vi "GermanInfo_Select_actual_values.vi"(11 "CSMinfo in":T1={"Общие сведения"={"Регистрационный номер заказа"="", "Идентификация (шифр) образца"="", "IMEI образца"="", "НД, устанавливающий требования"="", "Методы испытаний (измерений)"="", "Дата начала испытаний"="", "Дата завершения испытаний"=""}, "Климатические условия внешней среды"={"Температура окружающего воздуха"="", "Относительная влажность воздуха"="", "Атмосферное давление"=""}, "Окно с настройками"={"Режим звонка связь"=0, "Напряжение источника"=0, "Условия окружающей среды"=0, "Номер образца"=0, "Источник питания"=0, "Номер испытания"=0, "Режим звонка тональный модем"=0, "Количество итераций TM"=100.0, "Аутентификация"=0, "Колличество повторов измерений"=1.0, "Сим карта"=0, "VISA adress of CMW500"="", "Input attenuation"=1.0, "Output attenuation"=1.0, "Call Release Type"=0, "GSM Band"=0, "BCCH Channel Number"=0.0, "TCH Channel Number"=0.0, "Codec"=0, "AWGN"=0, "snrRatioInDb"=0.0, "GSM Fading"=0, "UL C/I ratio"=0, "Use a custom network ID"=FALSE, "MCC (Mobile Country Code)"=0.0, "MNC (Mobile Network Code)"=0.0, "NCC (Network Color Code)"=0.0, "MNC digit count"=0, "BCC (Base station Color Code)"=0.0, "LAC (Location Area Code)"=0.0, "RAC (Routing Area Code)"=0.0, "Cell Identity"=0.0, "Override UE ID"=FALSE, "MCC (UE Mobile Country Code)"=0.0, "MNC (UE Mobile Network Code)"=0.0, "MSIN (Mobile Subscription ID)"=0.0, "InputScaleFactor"=0, "OutputScaleFactor"=0, "Post MSD wave file playback 3GPP  26.269 \nEU_DTMF_tones"=FALSE, "Scenario"=0, "AlAckBehavior"=0, "PSAP listens for PUSH"=FALSE, "BCCH Channel Power"=0.0, "TCH Channel Power"=0.0, "Setting Path"=path "", "Алгоритм дозвона"=0}} {"Окно с настройками"."Алгоритм дозвона" items=["Standart", "Recall"]; "Окно с настройками"."AlAckBehavior" items=["POSITIVE", "CLEAR_DOWN", "LOOP_BACK_MSD_PART"]; "Окно с настройками"."Scenario" items=["NORMAL", "NORMAL_IMMEDIATE_START", "TIMEOUT_T3", "ALLRV_REQ", "SUPPRESS_MSD", "SUPPRESS_ALACK", "SUPPRESS_SEND_MSD"]; "Окно с настройками"."OutputScaleFactor" items=["ONE", "QUARTER", "HALF", "TWO", "FOUR"]; "Окно с настройками"."InputScaleFactor" items=["ONE", "QUARTER", "HALF", "TWO", "FOUR"]; "Окно с настройками"."MNC digit count" items=["TWO", "THREE"]; "Окно с настройками"."UL C/I ratio" items=["Ci1Db", "Ci4Db", "Ci7Db", "Ci10Db", "Ci13Db", "Ci16Db"]; "Окно с настройками"."GSM Fading" items=["GsmFadingOff", "GsmEtsiTs103412DlFading", "GsmEtsiTs103412UlFading", "GsmEtsiTs103412DlUlFading"]; "Окно с настройками"."AWGN" items=["Off", "50MhzAwgn"]; "Окно с настройками"."Codec" items=["FRV2", "AMRH_GMSK_7K95", "AMRH_GMSK_7K40", "AMRH_GMSK_6K70", "AMRH_GMSK_5K90", "AMRH_GMSK_5K15", "AMRH_GMSK_4K75", "AMRF_GMSK_12K20", "AMRF_GMSK_10K20", "AMRF_GMSK_7K95", "AMRF_GMSK_7K40 ", "AMRF_GMSK_6K70", "AMRF_GMSK_5K90", "AMRF_GMSK_5K15", "AMRF_GMSK_4K75", "FRV1", "HRV1", "WAMR_GMSK_6K60", "WAMR_GMSK_8K85", "WAMR_GMSK_12K65"]; "Окно с настройками"."GSM Band" items=["GSM450", "GSM850", "GSM900", "GSM1800", "GSM1900"]; "Окно с настройками"."Call Release Type" items=["NormalRelease", "CallInterruption"]; "Окно с настройками"."Сим карта" items=["SIM", "eSIM"]; "Окно с настройками"."Колличество повторов измерений" min=1.0 max=100.0 format="%#_3g"; "Окно с настройками"."Аутентификация" items=["On", "Off"]; "Окно с настройками"."Режим звонка тональный модем" items=["Автоматически (AT) GEMALTO", "Автоматически (AT) SIMCOM", "Автоматически (AT) SIMCOM SIM7600E-H", "Автоматически (AT) TELIT", "Автоматически (AT) PROGRESS", "Автоматически (AT) PROGRESS GREEN", "Автоматически (AT) PROGRESS BLUE", "Автоматически (реле)", "Вручную"]; "Окно с настройками"."Номер испытания" items=["1", "2", "3"]; "Окно с настройками"."Источник питания" items=["Не используется", "IT6332A"]; "Окно с настройками"."Номер образца" items=["1", "2", "3"]; "Окно с настройками"."Условия окружающей среды" items=["UnormTnorm", "UminTmin", "UmaxTmin", "UminTmax", "UmaxTmax", "TypeA", "TypeB"]; "Окно с настройками"."Напряжение источника" items=["12", "24"]; "Окно с настройками"."Режим звонка связь" items=["Автоматически (AT) GEMALTO", "Автоматически (AT) SIMCOM", "Автоматически (AT) SIMCOM SIM7600E-H", "Автоматически (AT) TELIT", "Автоматически (AT) PROGRESS", "Автоматически (AT) PROGRESS GREEN", "Автоматически (AT) PROGRESS BLUE", "Автоматически (реле)", "Вручную"]}) -> (0 "Условия окружающей среды":u16, 1 "Напряжение источника":u16, 2 "Образец":u16, 3 "Режим звонка":u16)   [LabVIEW 2018]
uses:
  CSM MOSCOW/CSMinfo/data/CSMinfo.ctl
panel:
  # "1. Общие настройки"
  # "Настройки модема по умолчанию"
  # "CMW500"
  # "PSAP"
  # "8.6.6"
  # "8.6.7"
  # "GSM"
  # "2. Настройки связи"
  # "8.6.8 (Use parameter NORMAL_IMMEDIATE_START)"
  # "8.6.9 (Use parameter LOOP_BACK_MSD_PART)"
  # "8.6.6"
  # "3. Настройки тонального модема"
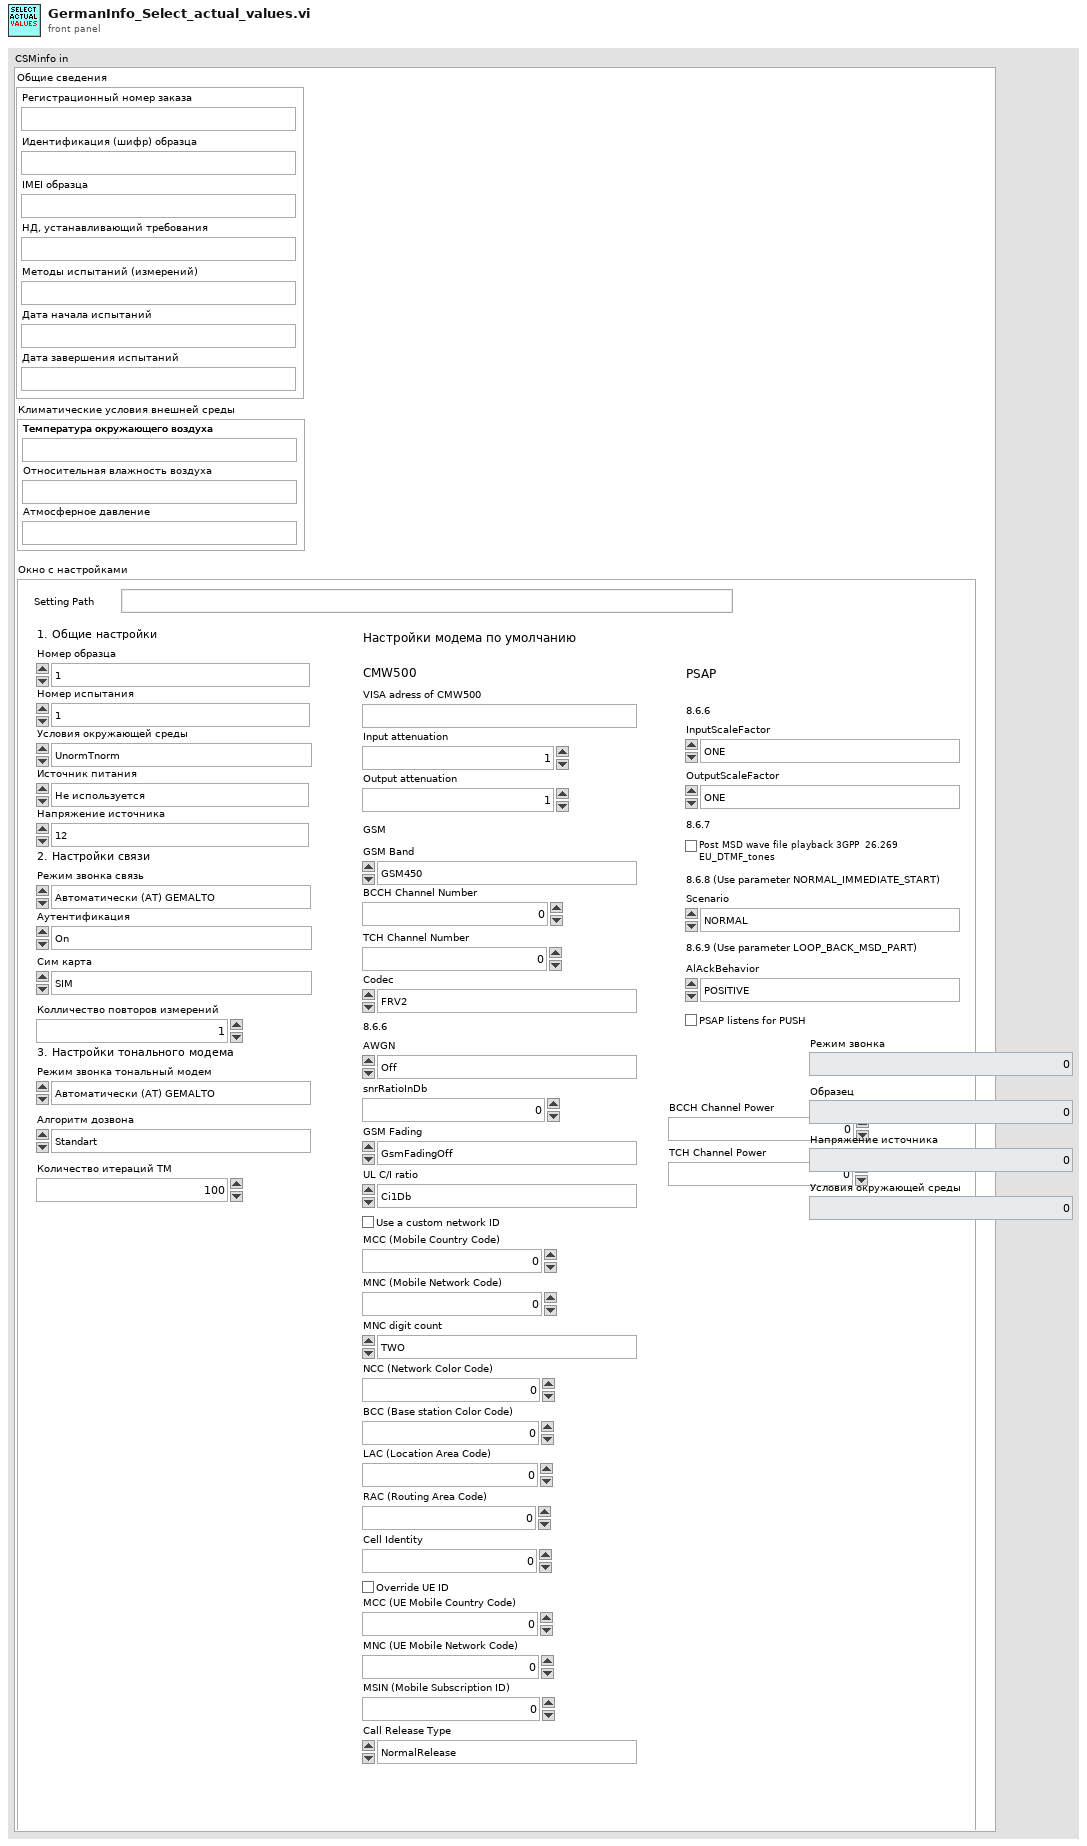
[diagram p1: front panel]
types:
  T1 = typedef "CSMinfo.ctl" = cluster{"Общие сведения":cluster{"Регистрационный номер заказа":string, "Идентификация (шифр) образца":string, "IMEI образца":string, "НД, устанавливающий требования":string, "Методы испытаний (измерений)":string, "Дата начала испытаний":string, "Дата завершения испытаний":string}, "Климатические условия внешней среды":cluster{"Температура окружающего воздуха":string, "Относительная влажность воздуха":string, "Атмосферное давление":string}, "Окно с настройками":cluster{"Режим звонка связь":u16, "Напряжение источника":u16, "Условия окружающей среды":u16, "Номер образца":u16, "Источник питания":u16, "Номер испытания":u16, "Режим звонка тональный модем":u16, "Количество итераций TM":dbl, "Аутентификация":u16, "Колличество повторов измерений":dbl, "Сим карта":u16, "VISA adress of CMW500":string, "Input attenuation":dbl, "Output attenuation":dbl, "Call Release Type":u16, "GSM Band":u16, "BCCH Channel Number":dbl, "TCH Channel Number":dbl, "Codec":u16, "AWGN":u16, "snrRatioInDb":dbl, "GSM Fading":u16, "UL C/I ratio":u16, "Use a custom network ID":bool, "MCC (Mobile Country Code)":dbl, "MNC (Mobile Network Code)":dbl, "NCC (Network Color Code)":dbl, "MNC digit count":u16, "BCC (Base station Color Code)":dbl, "LAC (Location Area Code)":dbl, "RAC (Routing Area Code)":dbl, "Cell Identity":dbl, "Override UE ID":bool, "MCC (UE Mobile Country Code)":dbl, "MNC (UE Mobile Network Code)":dbl, "MSIN (Mobile Subscription ID)":dbl, "InputScaleFactor":u16, "OutputScaleFactor":u16, "Post MSD wave file playback 3GPP  26.269 \nEU_DTMF_tones":bool, "Scenario":u16, "AlAckBehavior":u16, "PSAP listens for PUSH":bool, "BCCH Channel Power":dbl, "TCH Channel Power":dbl, "Setting Path":path, "Алгоритм дозвона":u16}}
  T2 = cluster{"Режим звонка связь":u16, "Напряжение источника":u16, "Условия окружающей среды":u16, "Номер образца":u16, "Источник питания":u16, "Номер испытания":u16, "Режим звонка тональный модем":u16, "Количество итераций TM":dbl, "Аутентификация":u16, "Колличество повторов измерений":dbl, "Сим карта":u16, "VISA adress of CMW500":string, "Input attenuation":dbl, "Output attenuation":dbl, "Call Release Type":u16, "GSM Band":u16, "BCCH Channel Number":dbl, "TCH Channel Number":dbl, "Codec":u16, "AWGN":u16, "snrRatioInDb":dbl, "GSM Fading":u16, "UL C/I ratio":u16, "Use a custom network ID":bool, "MCC (Mobile Country Code)":dbl, "MNC (Mobile Network Code)":dbl, "NCC (Network Color Code)":dbl, "MNC digit count":u16, "BCC (Base station Color Code)":dbl, "LAC (Location Area Code)":dbl, "RAC (Routing Area Code)":dbl, "Cell Identity":dbl, "Override UE ID":bool, "MCC (UE Mobile Country Code)":dbl, "MNC (UE Mobile Network Code)":dbl, "MSIN (Mobile Subscription ID)":dbl, "InputScaleFactor":u16, "OutputScaleFactor":u16, "Post MSD wave file playback 3GPP  26.269 \nEU_DTMF_tones":bool, "Scenario":u16, "AlAckBehavior":u16, "PSAP listens for PUSH":bool, "BCCH Channel Power":dbl, "TCH Channel Power":dbl, "Setting Path":path, "Алгоритм дозвона":u16}
  T3 = typedef "LVStringsAndValuesArrayTypeDef_U16.ctl" = cluster{"String":string, "Value":u16}[]
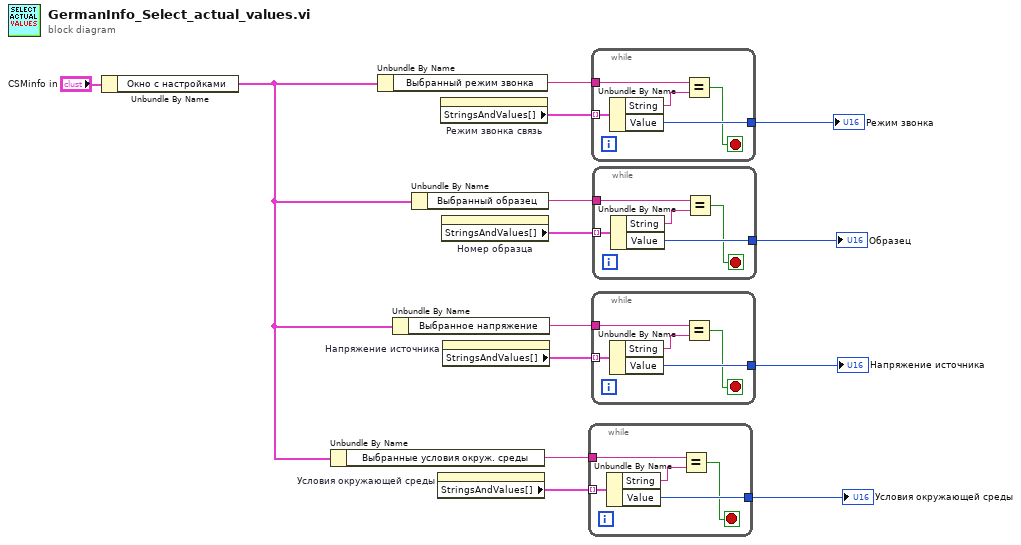
[diagram p0: block diagram]
diagram:
  n1 = Unbundle By Name("CSMinfo in") -> ("Окно с настройками"=w5:T2)
  n2 = Unbundle By Name(w5) -> ("Выбранные условия окруж. среды"=w8:string)
  n3 = Unbundle By Name(w5) -> ("Выбранный режим звонка"=w12:string)
  n4 = Unbundle By Name(w5) -> ("Выбранное напряжение"=w9:string)
  n5 = Unbundle By Name(w5) -> ("Выбранный образец"=w11:string)
  n6 = property on="Условия окружающей среды" class="Ring (strict)"() -> ("StringsAndValues[]"=w6:T3)  [unwired: 2 in, 2 out]
  n7 = property on="Режим звонка связь" class="Ring (strict)"() -> ("StringsAndValues[]"=w13:T3)  [unwired: 2 in, 2 out]
  n8 = property on="Номер образца" class="Ring (strict)"() -> ("StringsAndValues[]"=w10:T3)  [unwired: 2 in, 2 out]
  n9 = property on="Напряжение источника" class="Ring (strict)"() -> ("StringsAndValues[]"=w7:T3)  [unwired: 2 in, 2 out]
  n10 = while {
    tunnel: w6 -> [w19] mode=indexing
    tunnel: w8 -> [w18]
    tunnel: [w16] -> w1
    stop <- w15 stop-if-true
    n11 = Unbundle By Name(w19) -> ("String"=w17:string, "Value"=w16:u16)
    n12 = Equal?(x=w18, y=w17) -> (x = y?=w15:bool)
  }
  "Условия окружающей среды" <- w1
  n13 = while {
    tunnel: w13 -> [w24] mode=indexing
    tunnel: w12 -> [w23]
    tunnel: [w21] -> w4
    stop <- w20 stop-if-true
    n14 = Unbundle By Name(w24) -> ("String"=w22:string, "Value"=w21:u16)
    n15 = Equal?(x=w23, y=w22) -> (x = y?=w20:bool)
  }
  "Режим звонка" <- w4
  n16 = while {
    tunnel: w7 -> [w29] mode=indexing
    tunnel: w9 -> [w28]
    tunnel: [w26] -> w2
    stop <- w25 stop-if-true
    n17 = Unbundle By Name(w29) -> ("String"=w27:string, "Value"=w26:u16)
    n18 = Equal?(x=w28, y=w27) -> (x = y?=w25:bool)
  }
  "Напряжение источника" <- w2
  n19 = while {
    tunnel: w10 -> [w34] mode=indexing
    tunnel: w11 -> [w33]
    tunnel: [w31] -> w3
    stop <- w30 stop-if-true
    n20 = Unbundle By Name(w34) -> ("String"=w32:string, "Value"=w31:u16)
    n21 = Equal?(x=w33, y=w32) -> (x = y?=w30:bool)
  }
  "Образец" <- w3
